vi "Mapping Merge Live Data v10.2.1.vi"(0 "New Spectrum":T2, 1 "Target Position":T1={"Drive X Set"=10.0, "Drive Y Set"=10.0, "Drive Z Set"=10.0} {"Drive X Set" min=10.0 max=160.0 step=0.1 format="%.1f"; "Drive Z Set" min=10.0 max=160.0 step=0.1 format="%.1f"; "Drive Y Set" min=10.0 max=160.0 step=0.1 format="%.1f"}, 5 "X in (1D)":dbl[](array[numeric]), 7 "Y in (1D)":dbl[](array[numeric]), 9 "L in (2D)":dbl[][](array[numeric]), 11 "I in (2D)":dbl[][](array[numeric]), 12 "Step Size":dbl=1.0 caption="Step (µm)" min=0.1 max=30.0 step=0.1 format="%.1f") -> (4 "Live Data":dbl[][](array[numeric]), 6 "X out (1D)":dbl[](array[numeric]), 8 "Y out (1D)":dbl[](array[numeric]), 10 "L out (2D)":dbl[][](array[numeric]), 15 "I out (2D)":dbl[][](array[numeric]))   [LabVIEW 2010]
uses:
  NPC3SG/TypeDefs/NPC3SG Set Positions.ctl
panel:
  # "Target positions to provide equidistance for Raman Tool Set"
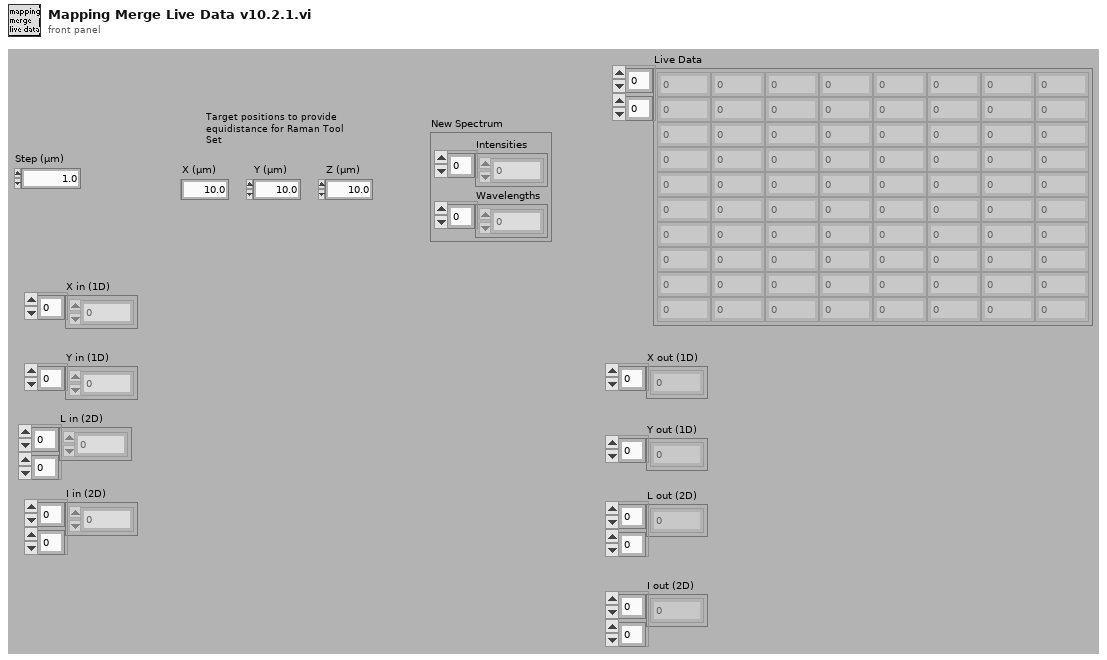
[diagram p1: front panel]
types:
  T1 = typedef "NPC3SG Set Positions.ctl" = cluster{"Drive X Set":dbl, "Drive Y Set":dbl, "Drive Z Set":dbl}
  T2 = cluster{"Wavelengths":dbl[], "Intensities":dbl[]}
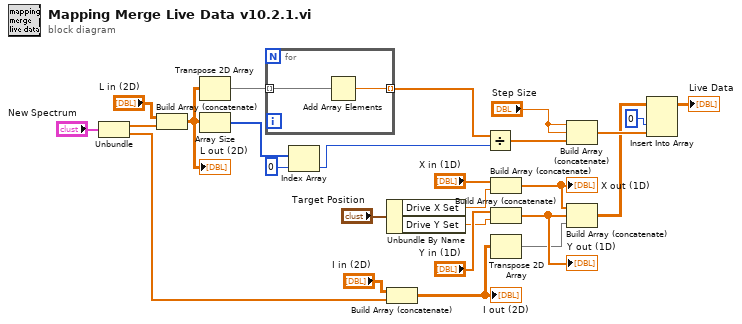
[diagram p0: block diagram]
diagram:
  n1 = Unbundle("New Spectrum") -> ("Wavelengths"=w26:dbl[], "Intensities"=w25:dbl[])
  n2 = Build Array (concatenate)("L in (2D)", w26) -> (w21:dbl[][])
  "L out (2D)" <- w21
  n3 = Transpose 2D Array(2D array=w21) -> (transposed array=w22:dbl[][])
  n4 = Array Size(array=w21) -> (size(s)=w14:i32[])
  n5 = for {
    tunnel: [w28] -> w12 mode=indexing
    tunnel: w22 -> [w27] mode=indexing
    n6 = Add Array Elements(numeric array=w27) -> (sum=w28:dbl)
  }
  n7 = Index Array(array=w14, index=0 ("Index")) -> (element=w16:i32)
  n8 = Unbundle By Name("Target Position") -> ("Drive X Set"=w7:dbl, "Drive Y Set"=w8:dbl)
  n9 = Build Array (concatenate)("I in (2D)", w25) -> (w20:dbl[][])
  "I out (2D)" <- w20
  n10 = Divide(x=w12, y=w16) -> (x/y=w13:dbl[])
  n11 = Build Array (concatenate)("X in (1D)", w7) -> (w18:dbl[])
  "X out (1D)" <- w18
  n12 = Build Array (concatenate)("Y in (1D)", w8) -> (w19:dbl[])
  "Y out (1D)" <- w19
  n13 = Transpose 2D Array(2D array=w20) -> (transposed array=w6:dbl[][])
  n14 = Build Array (concatenate)("Step Size", "Step Size", w13) -> (w5:dbl[])
  n15 = Build Array (concatenate)(w18, w19, w6) -> (w4:dbl[][])
  n16 = Insert Into Array(array=w4, index (col)=0 ("disabled index (col)"), new element=w5) -> (→"Live Data":dbl[][])  [unwired: 1 in]
